vi "SIM BDF resample BDs.vi"(3 "BDF data":T1, 4 "current stepSize":dbl, 5 "new stepSize":dbl) -> (0 "BDF data out":T1)   [LabVIEW 2010]
uses:
  SIM BDF data.ctl
  SIM Factored Matrix.ctl
  SIM BDF stages.ctl
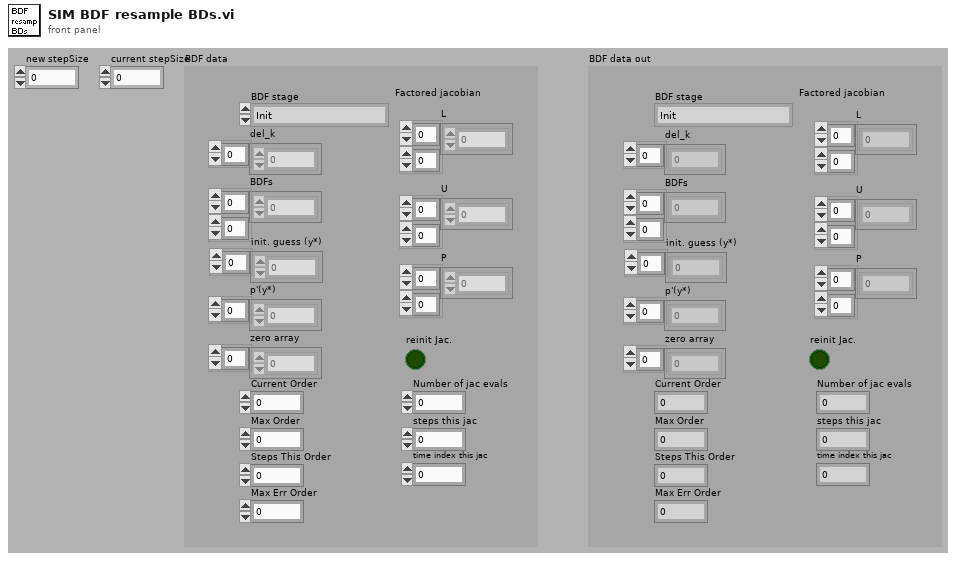
[diagram p1: front panel]
types:
  T1 = typedef "SIM BDF data.ctl" = cluster{"BDFs":dbl[][], "init. guess (y*)":dbl[], "p'(y*)":dbl[], "Factored jacobian":T2, "zero array":dbl[], "reinit Jac.":bool, "BDF stage":T3, "steps this jac":i32, "time index this jac":i32, "Number of jac evals":i32, "del_k":dbl[], "Current Order":i32, "Max Order":i32, "Steps This Order":i32, "Max Err Order":i32}
  T2 = typedef "SIM Factored Matrix.ctl" = cluster{"L":dbl[][], "U":dbl[][], "P":i32[][]}
  T3 = typedef "SIM BDF stages.ctl" = enum16{"Init", "Initial Guess", "Compute Jacobian", "Newton Iteration", "Eval Error", "Choose StepSize", "Reset BDFs"}
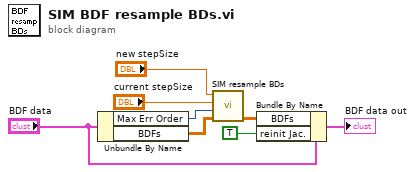
[diagram p0: block diagram]
diagram:
  n1 = Unbundle By Name("BDF data") -> ("Max Err Order"=w8:i32, "BDFs"=w1:dbl[][])
  n2 = call "SIM resample BDs.vi"("Backward differences"=w1, "interp poly order"=w8, "current timestep"="current stepSize", "new timestep"="new stepSize") -> ("New Backward differences"=w3:dbl[][])  [unwired: 7 out]
  n3 = Bundle By Name(cluster="BDF data", "BDFs"=w3, "reinit Jac."=TRUE) -> (→"BDF data out":T1)
